vi "ELVIS III v1.0 Reserve Channel.vi"(5 "Allow multiple opens?":bool, 7 "Owner":string, 8 "error in (no error)":errorcluster, 9 "Mutex IDs":u32[](array[numeric]), 10 "Connector":T1=enum."ConnectorB", 11 "Channel Name":string) -> (0 "error out":errorcluster)   [LabVIEW 2021]
uses:
  <vilib>/myRIO/Common/Instrument Driver Framework/ELVIS III v1.0/Resource Manager/typedefs/ELVIS III v1.0 Connector List.ctl
  <vilib>/myRIO/Common/Instrument Driver Framework/Utilities/typedefs/Resource Manager Action Enum.ctl
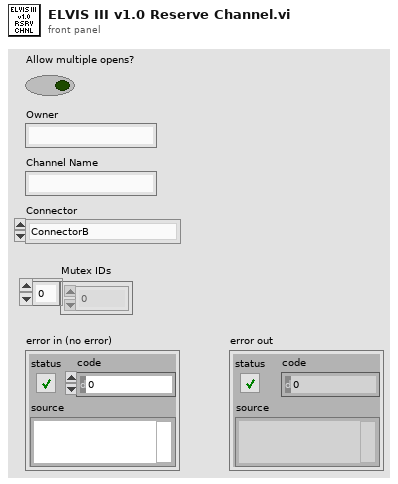
[diagram p1: front panel]
types:
  T1 = typedef "ELVIS III v1.0 Connector List.ctl" = enum32{"None", "ConnectorA", "ConnectorB"}
  T2 = typedef "Resource Manager Action Enum.ctl" = enum16{"Lock", "Unlock"}
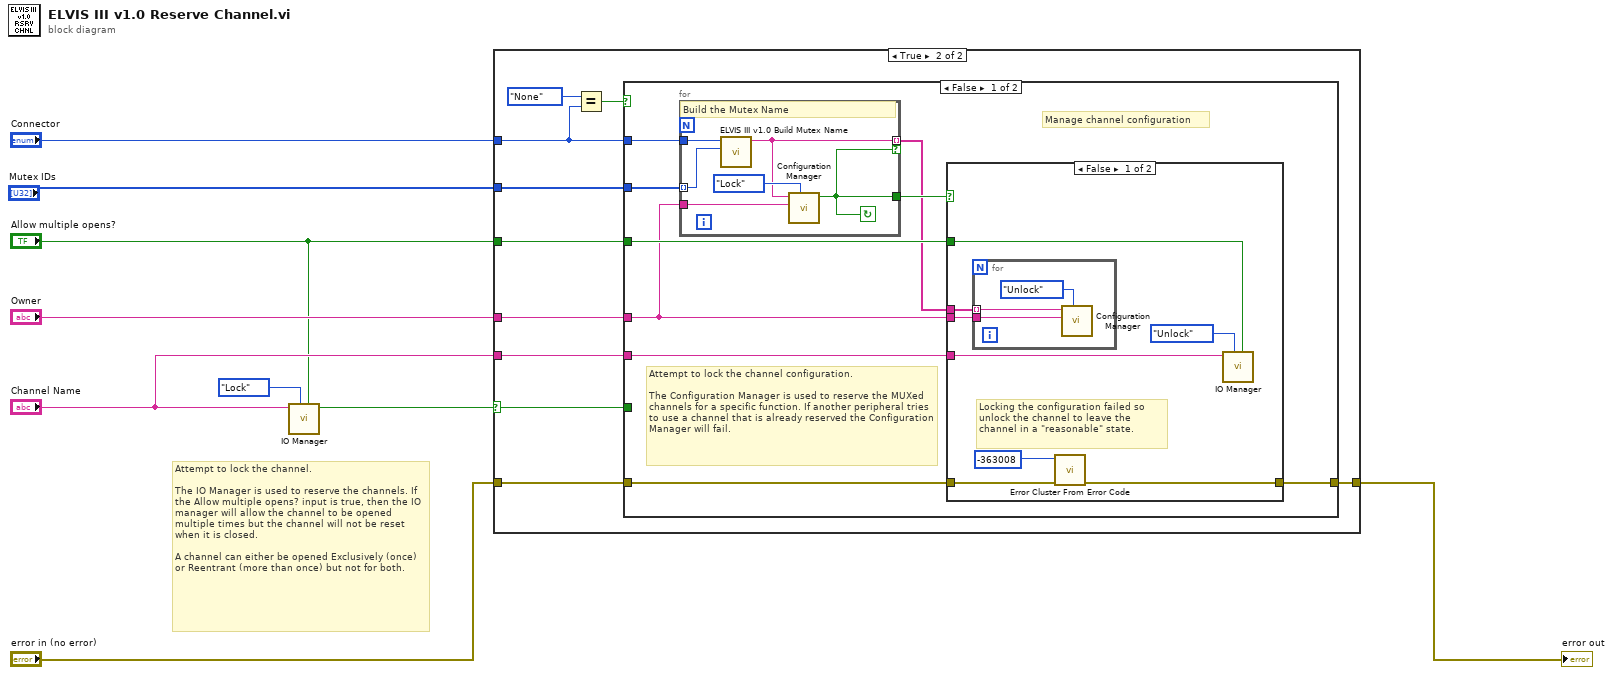
[diagram p0: block diagram]
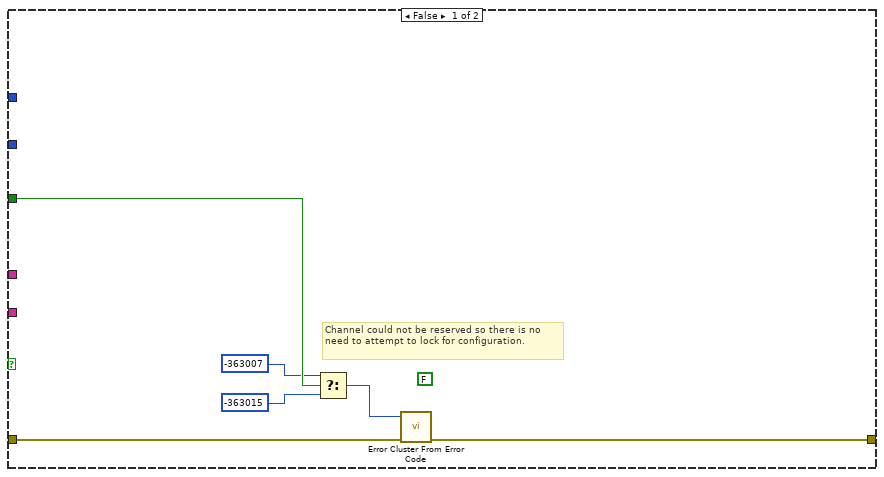
[diagram p2: hidden frame]
diagram:
  # "Attempt to lock the channel.\n\nThe IO Manager is used to reserve the channels. If the Allow multiple opens? input is true, then the IO manager will allow the channel to be opened multiple times but the channel will not be reset when it is closed.\n\nA channel can either be opened Exclusively (once) or Reentrant (more than once) but not for both."
  n1 = call <vilib>:"IO Manager.vi"("Reentrant?"="Allow multiple opens?", "Actions"=Resource_Manager_Action_Enum."Lock", "Mutex Name"="Channel Name") -> ("Success?"=w3:bool)  [unwired: 8 in]
  n2 = case shown="True" w3 {
    selector: w3 -> [_ w18]
    tunnel: "Channel Name" -> [_ w25]
    tunnel: "Owner" -> [_ w24]
    tunnel: "Allow multiple opens?" -> [w13 w23]
    tunnel: "Mutex IDs" -> [_ w22]
    tunnel: "Connector" -> [_ w21]
    tunnel: "error in (no error)" -> [w15 w17]
    tunnel: [w14 w16] -> w4
    frame False {
      (unwired) FALSE ("Reentrant?")
      # "Channel could not be reserved so there is no need to attempt to lock for configuration."
      n3 = Select(t=-363007 ("error code (0)"), s=w13, f=-363015 ("error code (0)")) -> (s? t:f=w11:i32)
      n4 = call <vilib>:"Error Cluster From Error Code.vi"("error in (no error)"=w15, "error code (0)"=w11) -> ("error out"=w14:errorcluster)  [unwired: 7 in]
    }
    frame True {
      n5 = Equal?(x=ELVIS_III_v1.0_Connector_List."None", y=w21) -> (x = y?=w19:bool)
      n6 = case shown="False" w19 {
        tunnel: w25 -> [w34 _]
        tunnel: w24 -> [w26 _]
        tunnel: w18 -> [_ _]
        tunnel: w23 -> [w33 _]
        tunnel: w21 -> [w28 _]
        tunnel: w22 -> [w32 _]
        tunnel: w17 -> [w30 w53]
        tunnel: [w29 w53] -> w16
        frame False {
          # "Attempt to lock the channel configuration.\n\nThe Configuration Manager is used to reserve the MUXed channels for a specific function. If another peripheral tries to use a channel that is already reserved the Configuration Manager will fail."
          # "Manage channel configuration"
          n7 = for {
            tunnel: w26 -> [w40]
            tunnel: w28 -> [w39]
            tunnel: w32 -> [w37] mode=indexing
            tunnel: [w36] -> w31
            tunnel: [w35] -> w27 mode=indexing if=w36
            stop <- w36 continue-if-true
            # "Build the Mutex Name"
            n8 = call <vilib>:"ELVIS III v1.0 Build Mutex Name.vi"("Mutex ID"=w37, "Connector"=w39) -> ("Mutex Name"=w35:string)  [unwired: 9 in]
            n9 = call <vilib>:"Configuration Manager.vi"("Actions"=Resource_Manager_Action_Enum."Lock", "Owner"=w40, "Mutex Name"=w35) -> ("Success?"=w36:bool)  [unwired: 8 in]
          }
          n10 = case shown="False" w31 {
            tunnel: w34 -> [w47 _]
            tunnel: w33 -> [w46 _]
            tunnel: w30 -> [w45 w52]
            tunnel: [w43 w52] -> w29
            tunnel: w27 -> [w42 _]
            tunnel: w26 -> [w41 _]
            frame False {
              # "Locking the configuration failed so unlock the channel to leave the channel in a \"reasonable\" state."
              n11 = for {
                tunnel: w42 -> [w49] mode=indexing
                tunnel: w41 -> [w50]
                n12 = call <vilib>:"Configuration Manager.vi"("Actions"=Resource_Manager_Action_Enum."Unlock", "Owner"=w50, "Mutex Name"=w49) -> ()  [unwired: 8 in, 1 out]
              }
              n13 = call <vilib>:"Error Cluster From Error Code.vi"("error in (no error)"=w45, "error code (0)"=-363008) -> ("error out"=w43:errorcluster)  [unwired: 7 in]
              n14 = call <vilib>:"IO Manager.vi"("Reentrant?"=w46, "Actions"=Resource_Manager_Action_Enum."Unlock", "Mutex Name"=w47) -> ()  [unwired: 8 in, 1 out]
            }
            frame True {
            }
          }
        }
        frame True {
          # "If there is no connector then there is no channel configuration to manage."
        }
      }
    }
  }
  "error out" <- w4
